vi "Read Remaining Length (bytes).vi"(11 "ControlPacket in":refnum<class "ControlPacket.lvclass">) -> (1 "Length":bool, 2 "Remaining Length (bytes)":u32, 3 "ControlPacket out":refnum<class "ControlPacket.lvclass">)   [LabVIEW 2013, in "ControlPacket.lvclass"]
uses:
  ControlPacket.lvclass
  ControlPacket.lvclass/ControlPacket.ctl
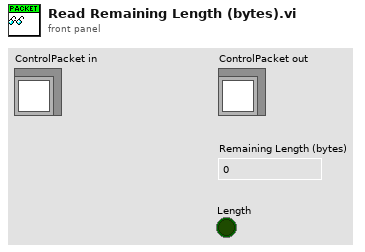
[diagram p1: front panel]
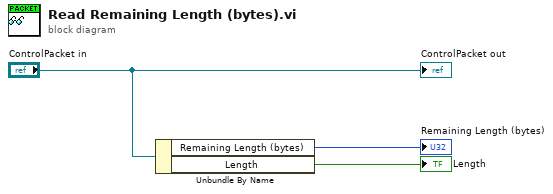
[diagram p0: block diagram]
diagram:
  n1 = Unbundle By Name("ControlPacket in") -> ("Remaining Length (bytes)"=→"Remaining Length (bytes)":u32, "Length"=→"Length":bool)
  "ControlPacket out" <- "ControlPacket in"
